vi "Multiplier4.vi"() -> (8 "Multiplier4":refnum<class "Multiplier4.lvclass">)   [LabVIEW 2017, in "Multiplier4.lvclass"]
uses:
  Multiplier4.lvclass
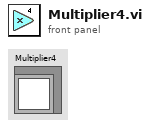
[diagram p1: front panel]
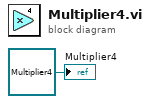
[diagram p0: block diagram]
diagram:
  "Multiplier4" <- refnum<class "Multiplier4.lvclass"> refnum ("Multiplier4.lvclass")
